vi "Configure Marker Search.vi"(0 "VISA resource name":refnum<visa-resource-name>, 1 "Search Range X (1: Full Range)":u16(ring)=1 items=["Band Marker X", "Full Range"], 2 "Peak Polarity (0: Positive)":enum16{"Positive", "Negative", "Both"}(ring), 3 "Target Transition (2: Both)":enum16{"Positive", "Negative", "Both"}(ring)=enum."Both", 5 "Measurement Type (6: Phase Noise)":u16(ring)=6 items=["AM Noise"=1, "Baseband Noise"=2, "Freq/Power"=3, "Spectrum"=4, "Transient"=5, "Phase Noise"=6, "User"=7], 7 "Select Trace (1: 1)":u16(ring)=1 items=["1"=1, "2"=2, "3"=3, "4"=4, "5"=5, "6"=6, "7"=7, "8"=8], 9 "Select Marker (1: 1)":u16(ring)=1 items=["1"=1, "2"=2, "3"=3, "4"=4, "5"=5, "6"=6, "7"=7, "8"=8, "9"=9, "10"=10], 11 "error in (no error)":errorcluster, 12 "Search Range Y (1: Full Range)":u16(ring)=1 items=["Band Marker Y", "Full Range"], 13 "Peak Excursion (0)":dbl format="%^#_9g", 14 "Target Value (0)":dbl format="%^#_9g") -> (4 "VISA resource name out":refnum<visa-resource-name>, 15 "error out":errorcluster)   [LabVIEW 2011, in "Agilent E5052X.lvlib"]
doc: "Sets the search properties for each marker in each trace.\n\n<b>Note: </b>\n\n \"Configure Marker\" VI must be run before this VI to enable markers before trying to configure their search settings."
uses:
  Agilent E5052X.lvlib
panel:
  # "Search Range Settings"
  # "Peak Search Settings"
  # "Target Search Settings"
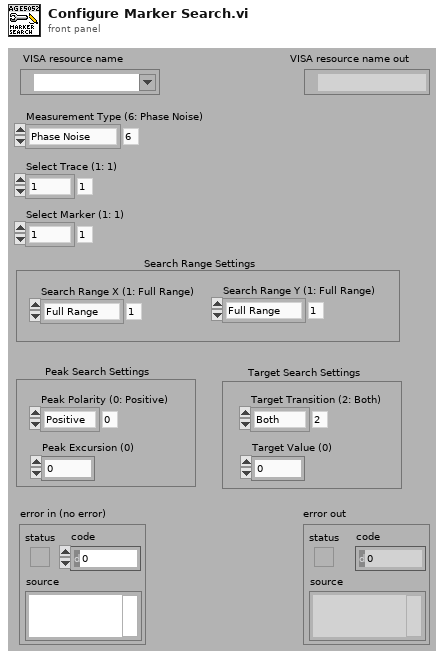
[diagram p1: front panel]
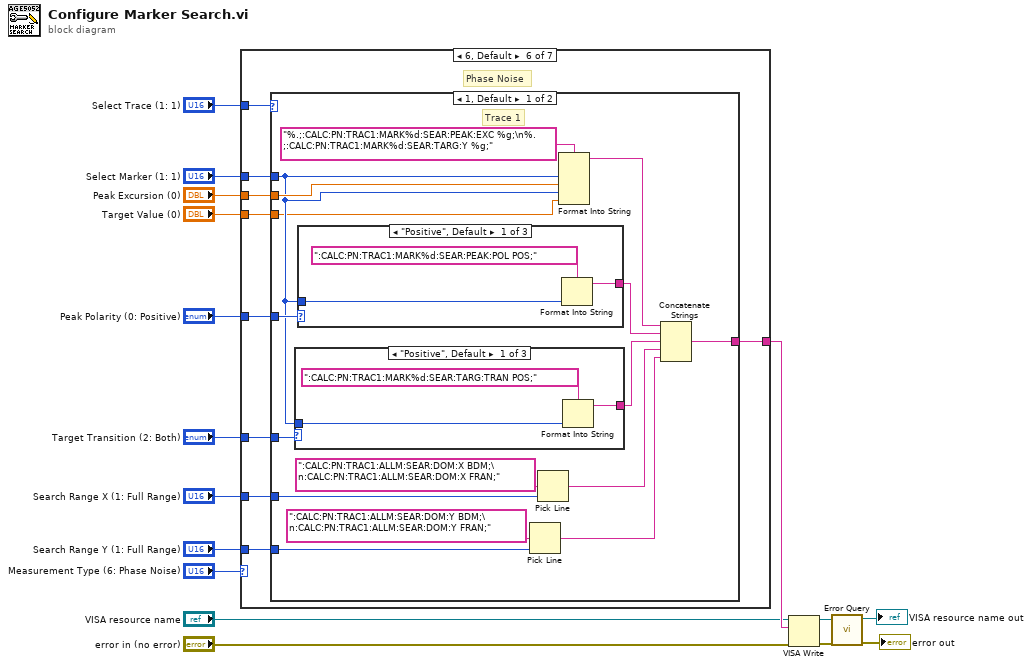
[diagram p0: block diagram]
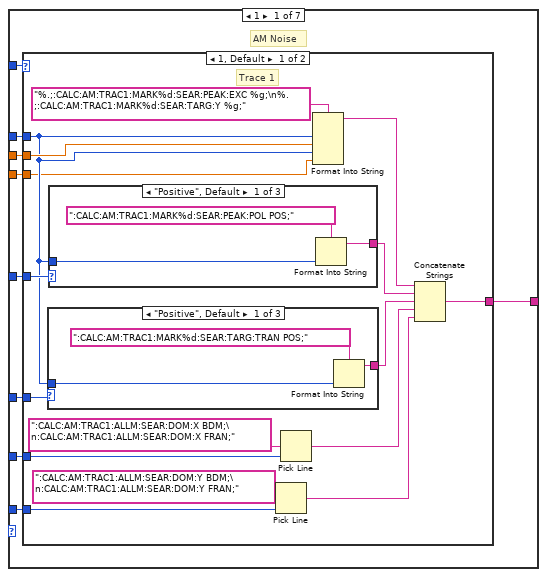
[diagram p2: hidden frame]
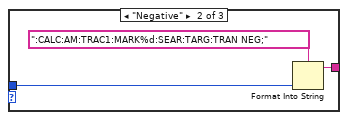
[diagram p3: hidden frame]
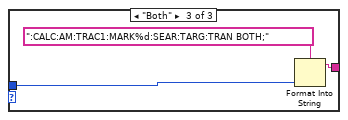
[diagram p4: hidden frame]
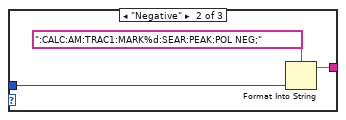
[diagram p5: hidden frame]
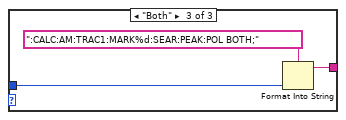
[diagram p6: hidden frame]
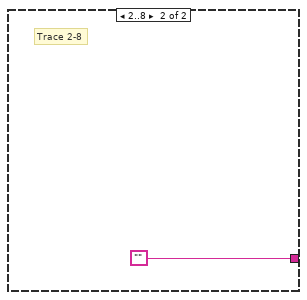
[diagram p7: hidden frame]
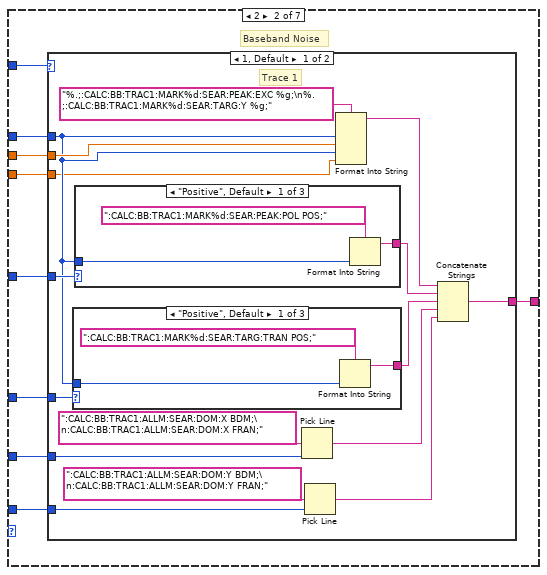
[diagram p8: hidden frame]
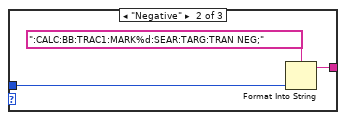
[diagram p9: hidden frame]
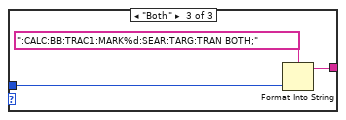
[diagram p10: hidden frame]
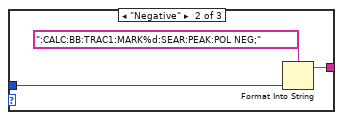
[diagram p11: hidden frame]
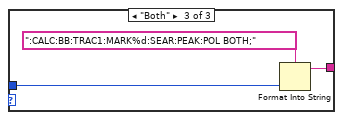
[diagram p12: hidden frame]
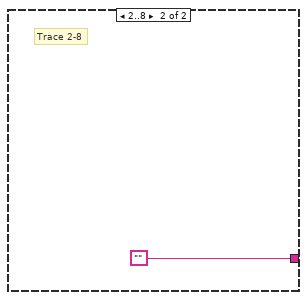
[diagram p13: hidden frame]
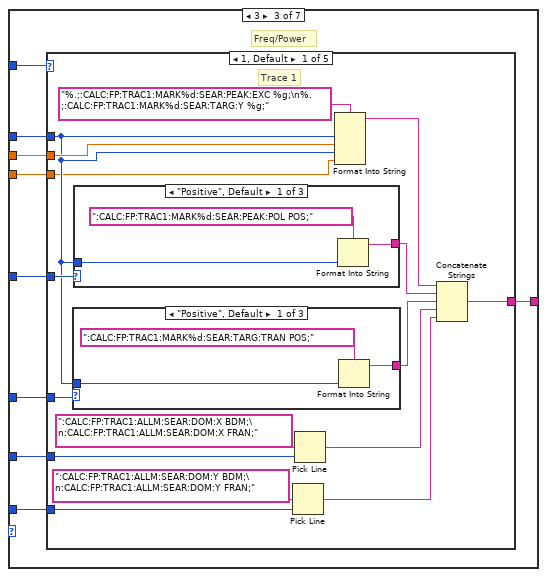
[diagram p14: hidden frame]
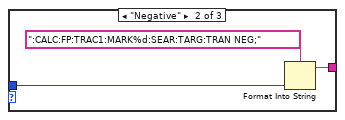
[diagram p15: hidden frame]
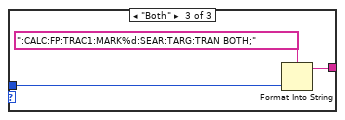
[diagram p16: hidden frame]
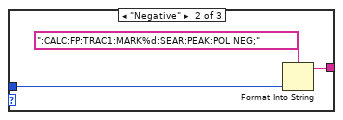
[diagram p17: hidden frame]
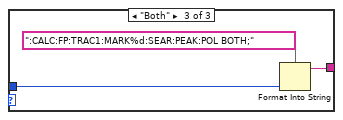
[diagram p18: hidden frame]
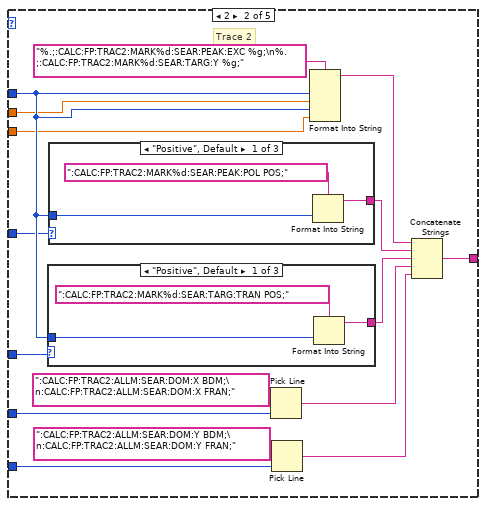
[diagram p19: hidden frame]
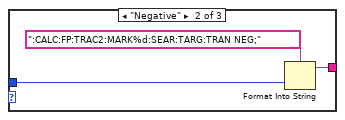
[diagram p20: hidden frame]
diagram:
  n1 = case shown="6, Default" "Measurement Type (6: Phase Noise)" {
    tunnel: "Select Marker (1: 1)" -> [w24 w68 w112 w258 w302 w448 w492]
    tunnel: "Select Trace (1: 1)" -> [w25 w69 w113 w259 w303 w449 w493]
    tunnel: "Search Range X (1: Full Range)" -> [w21 w63 w107 w253 w297 w443 w487]
    tunnel: "Search Range Y (1: Full Range)" -> [w20 w62 w106 w252 w296 w442 w486]
    tunnel: "Peak Excursion (0)" -> [w23 w67 w111 w257 w301 w447 w491]
    tunnel: "Peak Polarity (0: Positive)" -> [w22 w65 w109 w255 w299 w445 w489]
    tunnel: "Target Transition (2: Both)" -> [w19 w64 w108 w254 w298 w444 w488]
    tunnel: "Target Value (0)" -> [w18 w66 w110 w256 w300 w446 w490]
    tunnel: [w17 w61 w105 w251 w295 w441 w485] -> w8
    frame 1 {
      # "AM Noise"
      n2 = case shown="1, Default" w25 {
        tunnel: w24 -> [w37 _]
        tunnel: w23 -> [w40 _]
        tunnel: [w32 ""] -> w17
        tunnel: w22 -> [w39 _]
        tunnel: w21 -> [w30 _]
        tunnel: w20 -> [w27 _]
        tunnel: w19 -> [w38 _]
        tunnel: w18 -> [w36 _]
        frame 1, Default {
          # "Trace 1"
          n3 = case shown="\"Positive\", Default" w38 {
            tunnel: w37 -> [w44 w46 w49]
            tunnel: [w42 w45 w48] -> w33
            frame "Positive", Default {
              n4 = Format Into String(format string=":CALC:AM:TRAC1:MARK%d:SEAR:TARG:TRAN POS;", w44) -> (resulting string=w42:string)  [unwired: 2 in, 1 out]
            }
            frame "Negative" {
              n5 = Format Into String(format string=":CALC:AM:TRAC1:MARK%d:SEAR:TARG:TRAN NEG;", w46) -> (resulting string=w45:string)  [unwired: 2 in, 1 out]
            }
            frame "Both" {
              n6 = Format Into String(format string=":CALC:AM:TRAC1:MARK%d:SEAR:TARG:TRAN BOTH;", w49) -> (resulting string=w48:string)  [unwired: 2 in, 1 out]
            }
          }
          n7 = case shown="\"Positive\", Default" w39 {
            tunnel: w37 -> [w53 w55 w58]
            tunnel: [w51 w54 w57] -> w34
            frame "Positive", Default {
              n8 = Format Into String(format string=":CALC:AM:TRAC1:MARK%d:SEAR:PEAK:POL POS;", w53) -> (resulting string=w51:string)  [unwired: 2 in, 1 out]
            }
            frame "Negative" {
              n9 = Format Into String(format string=":CALC:AM:TRAC1:MARK%d:SEAR:PEAK:POL NEG;", w55) -> (resulting string=w54:string)  [unwired: 2 in, 1 out]
            }
            frame "Both" {
              n10 = Format Into String(format string=":CALC:AM:TRAC1:MARK%d:SEAR:PEAK:POL BOTH;", w58) -> (resulting string=w57:string)  [unwired: 2 in, 1 out]
            }
          }
          n11 = Pick Line(multi-line string=":CALC:AM:TRAC1:ALLM:SEAR:DOM:Y BDM;\n:CALC:AM:TRAC1:ALLM:SEAR:DOM:Y FRAN;", line index=w27) -> (output string=w26:string)  [unwired: 1 in]
          n12 = Pick Line(multi-line string=":CALC:AM:TRAC1:ALLM:SEAR:DOM:X BDM;\n:CALC:AM:TRAC1:ALLM:SEAR:DOM:X FRAN;", line index=w30) -> (output string=w29:string)  [unwired: 1 in]
          n13 = Format Into String(format string="%.;:CALC:AM:TRAC1:MARK%d:SEAR:PEAK:EXC %g;\n%.;:CALC:AM:TRAC1:MARK%d:SEAR:TARG:Y %g;", w37, w40, w37, w36) -> (resulting string=w35:string)  [unwired: 2 in, 1 out]
          n14 = Concatenate Strings(w35, w34, w33, w29, w26) -> (w32:string)
        }
        frame 2..8 {
          # "Trace 2-8"
        }
      }
    }
    frame 2 {
      # "Baseband Noise"
      n15 = case shown="1, Default" w69 {
        tunnel: w68 -> [w81 _]
        tunnel: w67 -> [w84 _]
        tunnel: [w76 ""] -> w61
        tunnel: w65 -> [w83 _]
        tunnel: w63 -> [w74 _]
        tunnel: w62 -> [w71 _]
        tunnel: w64 -> [w82 _]
        tunnel: w66 -> [w80 _]
        frame 1, Default {
          # "Trace 1"
          n16 = case shown="\"Positive\", Default" w82 {
            tunnel: w81 -> [w88 w90 w93]
            tunnel: [w86 w89 w92] -> w77
            frame "Positive", Default {
              n17 = Format Into String(format string=":CALC:BB:TRAC1:MARK%d:SEAR:TARG:TRAN POS;", w88) -> (resulting string=w86:string)  [unwired: 2 in, 1 out]
            }
            frame "Negative" {
              n18 = Format Into String(format string=":CALC:BB:TRAC1:MARK%d:SEAR:TARG:TRAN NEG;", w90) -> (resulting string=w89:string)  [unwired: 2 in, 1 out]
            }
            frame "Both" {
              n19 = Format Into String(format string=":CALC:BB:TRAC1:MARK%d:SEAR:TARG:TRAN BOTH;", w93) -> (resulting string=w92:string)  [unwired: 2 in, 1 out]
            }
          }
          n20 = case shown="\"Positive\", Default" w83 {
            tunnel: w81 -> [w97 w99 w102]
            tunnel: [w95 w98 w101] -> w78
            frame "Positive", Default {
              n21 = Format Into String(format string=":CALC:BB:TRAC1:MARK%d:SEAR:PEAK:POL POS;", w97) -> (resulting string=w95:string)  [unwired: 2 in, 1 out]
            }
            frame "Negative" {
              n22 = Format Into String(format string=":CALC:BB:TRAC1:MARK%d:SEAR:PEAK:POL NEG;", w99) -> (resulting string=w98:string)  [unwired: 2 in, 1 out]
            }
            frame "Both" {
              n23 = Format Into String(format string=":CALC:BB:TRAC1:MARK%d:SEAR:PEAK:POL BOTH;", w102) -> (resulting string=w101:string)  [unwired: 2 in, 1 out]
            }
          }
          n24 = Pick Line(multi-line string=":CALC:BB:TRAC1:ALLM:SEAR:DOM:X BDM;\n:CALC:BB:TRAC1:ALLM:SEAR:DOM:X FRAN;", line index=w74) -> (output string=w73:string)  [unwired: 1 in]
          n25 = Pick Line(multi-line string=":CALC:BB:TRAC1:ALLM:SEAR:DOM:Y BDM;\n:CALC:BB:TRAC1:ALLM:SEAR:DOM:Y FRAN;", line index=w71) -> (output string=w70:string)  [unwired: 1 in]
          n26 = Format Into String(format string="%.;:CALC:BB:TRAC1:MARK%d:SEAR:PEAK:EXC %g;\n%.;:CALC:BB:TRAC1:MARK%d:SEAR:TARG:Y %g;", w81, w84, w81, w80) -> (resulting string=w79:string)  [unwired: 2 in, 1 out]
          n27 = Concatenate Strings(w79, w78, w77, w73, w70) -> (w76:string)
        }
        frame 2..8 {
          # "Trace 2-8"
        }
      }
    }
    frame 3 {
      # "Freq/Power"
      n28 = case shown="1, Default" w113 {
        tunnel: w112 -> [w125 w159 w193 w227 _]
        tunnel: w111 -> [w128 w158 w192 w226 _]
        tunnel: [w120 w154 w188 w222 ""] -> w105
        tunnel: w109 -> [w127 w156 w190 w224 _]
        tunnel: w107 -> [w118 w152 w186 w220 _]
        tunnel: w106 -> [w115 w149 w183 w217 _]
        tunnel: w108 -> [w126 w155 w189 w223 _]
        tunnel: w110 -> [w124 w157 w191 w225 _]
        frame 1, Default {
          # "Trace 1"
          n29 = case shown="\"Positive\", Default" w126 {
            tunnel: w125 -> [w132 w134 w137]
            tunnel: [w130 w133 w136] -> w121
            frame "Positive", Default {
              n30 = Format Into String(format string=":CALC:FP:TRAC1:MARK%d:SEAR:TARG:TRAN POS;", w132) -> (resulting string=w130:string)  [unwired: 2 in, 1 out]
            }
            frame "Negative" {
              n31 = Format Into String(format string=":CALC:FP:TRAC1:MARK%d:SEAR:TARG:TRAN NEG;", w134) -> (resulting string=w133:string)  [unwired: 2 in, 1 out]
            }
            frame "Both" {
              n32 = Format Into String(format string=":CALC:FP:TRAC1:MARK%d:SEAR:TARG:TRAN BOTH;", w137) -> (resulting string=w136:string)  [unwired: 2 in, 1 out]
            }
          }
          n33 = case shown="\"Positive\", Default" w127 {
            tunnel: w125 -> [w141 w143 w146]
            tunnel: [w139 w142 w145] -> w122
            frame "Positive", Default {
              n34 = Format Into String(format string=":CALC:FP:TRAC1:MARK%d:SEAR:PEAK:POL POS;", w141) -> (resulting string=w139:string)  [unwired: 2 in, 1 out]
            }
            frame "Negative" {
              n35 = Format Into String(format string=":CALC:FP:TRAC1:MARK%d:SEAR:PEAK:POL NEG;", w143) -> (resulting string=w142:string)  [unwired: 2 in, 1 out]
            }
            frame "Both" {
              n36 = Format Into String(format string=":CALC:FP:TRAC1:MARK%d:SEAR:PEAK:POL BOTH;", w146) -> (resulting string=w145:string)  [unwired: 2 in, 1 out]
            }
          }
          n37 = Pick Line(multi-line string=":CALC:FP:TRAC1:ALLM:SEAR:DOM:Y BDM;\n:CALC:FP:TRAC1:ALLM:SEAR:DOM:Y FRAN;", line index=w115) -> (output string=w114:string)  [unwired: 1 in]
          n38 = Pick Line(multi-line string=":CALC:FP:TRAC1:ALLM:SEAR:DOM:X BDM;\n:CALC:FP:TRAC1:ALLM:SEAR:DOM:X FRAN;", line index=w118) -> (output string=w117:string)  [unwired: 1 in]
          n39 = Format Into String(format string="%.;:CALC:FP:TRAC1:MARK%d:SEAR:PEAK:EXC %g;\n%.;:CALC:FP:TRAC1:MARK%d:SEAR:TARG:Y %g;", w125, w128, w125, w124) -> (resulting string=w123:string)  [unwired: 2 in, 1 out]
          n40 = Concatenate Strings(w123, w122, w121, w117, w114) -> (w120:string)
        }
        frame 2 {
          # "Trace 2"
          n41 = case shown="\"Positive\", Default" w155 {
            tunnel: w159 -> [w166 w168 w171]
            tunnel: [w164 w167 w170] -> w160
            frame "Positive", Default {
              n42 = Format Into String(format string=":CALC:FP:TRAC2:MARK%d:SEAR:TARG:TRAN POS;", w166) -> (resulting string=w164:string)  [unwired: 2 in, 1 out]
            }
            frame "Negative" {
              n43 = Format Into String(format string=":CALC:FP:TRAC2:MARK%d:SEAR:TARG:TRAN NEG;", w168) -> (resulting string=w167:string)  [unwired: 2 in, 1 out]
            }
            frame "Both" {
              n44 = Format Into String(format string=":CALC:FP:TRAC2:MARK%d:SEAR:TARG:TRAN BOTH;", w171) -> (resulting string=w170:string)  [unwired: 2 in, 1 out]
            }
          }
          n45 = case shown="\"Positive\", Default" w156 {
            tunnel: w159 -> [w175 w177 w180]
            tunnel: [w173 w176 w179] -> w161
            frame "Positive", Default {
              n46 = Format Into String(format string=":CALC:FP:TRAC2:MARK%d:SEAR:PEAK:POL POS;", w175) -> (resulting string=w173:string)  [unwired: 2 in, 1 out]
            }
            frame "Negative" {
              n47 = Format Into String(format string=":CALC:FP:TRAC2:MARK%d:SEAR:PEAK:POL NEG;", w177) -> (resulting string=w176:string)  [unwired: 2 in, 1 out]
            }
            frame "Both" {
              n48 = Format Into String(format string=":CALC:FP:TRAC2:MARK%d:SEAR:PEAK:POL BOTH;", w180) -> (resulting string=w179:string)  [unwired: 2 in, 1 out]
            }
          }
          n49 = Pick Line(multi-line string=":CALC:FP:TRAC2:ALLM:SEAR:DOM:X BDM;\n:CALC:FP:TRAC2:ALLM:SEAR:DOM:X FRAN;", line index=w152) -> (output string=w151:string)  [unwired: 1 in]
          n50 = Pick Line(multi-line string=":CALC:FP:TRAC2:ALLM:SEAR:DOM:Y BDM;\n:CALC:FP:TRAC2:ALLM:SEAR:DOM:Y FRAN;", line index=w149) -> (output string=w148:string)  [unwired: 1 in]
          n51 = Format Into String(format string="%.;:CALC:FP:TRAC2:MARK%d:SEAR:PEAK:EXC %g;\n%.;:CALC:FP:TRAC2:MARK%d:SEAR:TARG:Y %g;", w159, w158, w159, w157) -> (resulting string=w162:string)  [unwired: 2 in, 1 out]
          n52 = Concatenate Strings(w162, w161, w160, w151, w148) -> (w154:string)
        }
        frame 3 {
          # "Trace 3"
          n53 = case shown="\"Both\"" w189 {
            tunnel: w193 -> [w200 w202 w205]
            tunnel: [w198 w201 w204] -> w194
            frame "Positive", Default {
              n54 = Format Into String(format string=":CALC:FP:TRAC3:MARK%d:SEAR:TARG:TRAN POS;", w200) -> (resulting string=w198:string)  [unwired: 2 in, 1 out]
            }
            frame "Negative" {
              n55 = Format Into String(format string=":CALC:FP:TRAC3:MARK%d:SEAR:TARG:TRAN NEG;", w202) -> (resulting string=w201:string)  [unwired: 2 in, 1 out]
            }
            frame "Both" {
              n56 = Format Into String(format string=":CALC:FP:TRAC3:MARK%d:SEAR:TARG:TRAN BOTH;", w205) -> (resulting string=w204:string)  [unwired: 2 in, 1 out]
            }
          }
          n57 = case shown="\"Positive\", Default" w190 {
            tunnel: w193 -> [w209 w211 w214]
            tunnel: [w207 w210 w213] -> w195
            frame "Positive", Default {
              n58 = Format Into String(format string=":CALC:FP:TRAC3:MARK%d:SEAR:PEAK:POL POS;", w209) -> (resulting string=w207:string)  [unwired: 2 in, 1 out]
            }
            frame "Negative" {
              n59 = Format Into String(format string=":CALC:FP:TRAC3:MARK%d:SEAR:PEAK:POL NEG;", w211) -> (resulting string=w210:string)  [unwired: 2 in, 1 out]
            }
            frame "Both" {
              n60 = Format Into String(format string=":CALC:FP:TRAC3:MARK%d:SEAR:PEAK:POL BOTH;", w214) -> (resulting string=w213:string)  [unwired: 2 in, 1 out]
            }
          }
          n61 = Pick Line(multi-line string=":CALC:FP:TRAC3:ALLM:SEAR:DOM:X BDM;\n:CALC:FP:TRAC3:ALLM:SEAR:DOM:X FRAN;", line index=w186) -> (output string=w185:string)  [unwired: 1 in]
          n62 = Pick Line(multi-line string=":CALC:FP:TRAC3:ALLM:SEAR:DOM:Y BDM;\n:CALC:FP:TRAC3:ALLM:SEAR:DOM:Y FRAN;", line index=w183) -> (output string=w182:string)  [unwired: 1 in]
          n63 = Format Into String(format string="%.;:CALC:FP:TRAC3:MARK%d:SEAR:PEAK:EXC %g;\n%.;:CALC:FP:TRAC3:MARK%d:SEAR:TARG:Y %g;", w193, w192, w193, w191) -> (resulting string=w196:string)  [unwired: 2 in, 1 out]
          n64 = Concatenate Strings(w196, w195, w194, w185, w182) -> (w188:string)
        }
        frame 4 {
          # "Trace 4"
          n65 = case shown="\"Positive\", Default" w223 {
            tunnel: w227 -> [w234 w236 w239]
            tunnel: [w232 w235 w238] -> w228
            frame "Positive", Default {
              n66 = Format Into String(format string=":CALC:FP:TRAC4:MARK%d:SEAR:TARG:TRAN POS;", w234) -> (resulting string=w232:string)  [unwired: 2 in, 1 out]
            }
            frame "Negative" {
              n67 = Format Into String(format string=":CALC:FP:TRAC4:MARK%d:SEAR:TARG:TRAN NEG;", w236) -> (resulting string=w235:string)  [unwired: 2 in, 1 out]
            }
            frame "Both" {
              n68 = Format Into String(format string=":CALC:FP:TRAC4:MARK%d:SEAR:TARG:TRAN BOTH;", w239) -> (resulting string=w238:string)  [unwired: 2 in, 1 out]
            }
          }
          n69 = case shown="\"Both\"" w224 {
            tunnel: w227 -> [w243 w245 w248]
            tunnel: [w241 w244 w247] -> w229
            frame "Positive", Default {
              n70 = Format Into String(format string=":CALC:FP:TRAC4:MARK%d:SEAR:PEAK:POL POS;", w243) -> (resulting string=w241:string)  [unwired: 2 in, 1 out]
            }
            frame "Negative" {
              n71 = Format Into String(format string=":CALC:FP:TRAC4:MARK%d:SEAR:PEAK:POL NEG;", w245) -> (resulting string=w244:string)  [unwired: 2 in, 1 out]
            }
            frame "Both" {
              n72 = Format Into String(format string=":CALC:FP:TRAC4:MARK%d:SEAR:PEAK:POL BOTH;", w248) -> (resulting string=w247:string)  [unwired: 2 in, 1 out]
            }
          }
          n73 = Pick Line(multi-line string=":CALC:FP:TRAC4:ALLM:SEAR:DOM:Y BDM;\n:CALC:FP:TRAC4:ALLM:SEAR:DOM:Y FRAN;", line index=w217) -> (output string=w216:string)  [unwired: 1 in]
          n74 = Pick Line(multi-line string=":CALC:FP:TRAC4:ALLM:SEAR:DOM:X BDM;\n:CALC:FP:TRAC4:ALLM:SEAR:DOM:X FRAN;", line index=w220) -> (output string=w219:string)  [unwired: 1 in]
          n75 = Format Into String(format string="%.;:CALC:FP:TRAC4:MARK%d:SEAR:PEAK:EXC %g;\n%.;:CALC:FP:TRAC4:MARK%d:SEAR:TARG:Y %g;", w227, w226, w227, w225) -> (resulting string=w230:string)  [unwired: 2 in, 1 out]
          n76 = Concatenate Strings(w230, w229, w228, w219, w216) -> (w222:string)
        }
        frame 5..8 {
          # "Trace 5..8"
        }
      }
    }
    frame 4 {
      # "Spectrum Monitor"
      n77 = case shown="1, Default" w259 {
        tunnel: w258 -> [w271 _]
        tunnel: w257 -> [w274 _]
        tunnel: [w266 ""] -> w251
        tunnel: w255 -> [w273 _]
        tunnel: w253 -> [w264 _]
        tunnel: w252 -> [w261 _]
        tunnel: w254 -> [w272 _]
        tunnel: w256 -> [w270 _]
        frame 1, Default {
          # "Trace 1"
          n78 = case shown="\"Positive\", Default" w272 {
            tunnel: w271 -> [w278 w280 w283]
            tunnel: [w276 w279 w282] -> w267
            frame "Positive", Default {
              n79 = Format Into String(format string=":CALC:SP:TRAC1:MARK%d:SEAR:TARG:TRAN POS;", w278) -> (resulting string=w276:string)  [unwired: 2 in, 1 out]
            }
            frame "Negative" {
              n80 = Format Into String(format string=":CALC:SP:TRAC1:MARK%d:SEAR:TARG:TRAN NEG;", w280) -> (resulting string=w279:string)  [unwired: 2 in, 1 out]
            }
            frame "Both" {
              n81 = Format Into String(format string=":CALC:SP:TRAC1:MARK%d:SEAR:TARG:TRAN BOTH;", w283) -> (resulting string=w282:string)  [unwired: 2 in, 1 out]
            }
          }
          n82 = case shown="\"Positive\", Default" w273 {
            tunnel: w271 -> [w287 w289 w292]
            tunnel: [w285 w288 w291] -> w268
            frame "Positive", Default {
              n83 = Format Into String(format string=":CALC:SP:TRAC1:MARK%d:SEAR:PEAK:POL POS;", w287) -> (resulting string=w285:string)  [unwired: 2 in, 1 out]
            }
            frame "Negative" {
              n84 = Format Into String(format string=":CALC:SP:TRAC1:MARK%d:SEAR:PEAK:POL NEG;", w289) -> (resulting string=w288:string)  [unwired: 2 in, 1 out]
            }
            frame "Both" {
              n85 = Format Into String(format string=":CALC:SP:TRAC1:MARK%d:SEAR:PEAK:POL BOTH;", w292) -> (resulting string=w291:string)  [unwired: 2 in, 1 out]
            }
          }
          n86 = Pick Line(multi-line string=":CALC:SP:TRAC1:ALLM:SEAR:DOM:X BDM;\n:CALC:SP:TRAC1:ALLM:SEAR:DOM:X FRAN;", line index=w264) -> (output string=w263:string)  [unwired: 1 in]
          n87 = Pick Line(multi-line string=":CALC:SP:TRAC1:ALLM:SEAR:DOM:Y BDM;\n:CALC:SP:TRAC1:ALLM:SEAR:DOM:Y FRAN;", line index=w261) -> (output string=w260:string)  [unwired: 1 in]
          n88 = Format Into String(format string="%.;:CALC:SP:TRAC1:MARK%d:SEAR:PEAK:EXC %g;\n%.;:CALC:SP:TRAC1:MARK%d:SEAR:TARG:Y %g;", w271, w274, w271, w270) -> (resulting string=w269:string)  [unwired: 2 in, 1 out]
          n89 = Concatenate Strings(w269, w268, w267, w263, w260) -> (w266:string)
        }
        frame 2..8 {
          # "Trace 2..8"
        }
      }
    }
    frame 5 {
      # "Transient"
      n90 = case shown="1, Default" w303 {
        tunnel: w302 -> [w315 w349 w383 w417 _]
        tunnel: w301 -> [w318 w348 w382 w416 _]
        tunnel: [w310 w344 w378 w412 ""] -> w295
        tunnel: w299 -> [w317 w346 w380 w414 _]
        tunnel: w297 -> [w308 w342 w376 w410 _]
        tunnel: w296 -> [w305 w339 w373 w407 _]
        tunnel: w298 -> [w316 w345 w379 w413 _]
        tunnel: w300 -> [w314 w347 w381 w415 _]
        frame 1, Default {
          # "Trace 1"
          n91 = case shown="\"Positive\", Default" w316 {
            tunnel: w315 -> [w322 w324 w327]
            tunnel: [w320 w323 w326] -> w311
            frame "Positive", Default {
              n92 = Format Into String(format string=":CALC:TR:TRAC1:MARK%d:SEAR:TARG:TRAN POS;", w322) -> (resulting string=w320:string)  [unwired: 2 in, 1 out]
            }
            frame "Negative" {
              n93 = Format Into String(format string=":CALC:TR:TRAC1:MARK%d:SEAR:TARG:TRAN NEG;", w324) -> (resulting string=w323:string)  [unwired: 2 in, 1 out]
            }
            frame "Both" {
              n94 = Format Into String(format string=":CALC:TR:TRAC1:MARK%d:SEAR:TARG:TRAN BOTH;", w327) -> (resulting string=w326:string)  [unwired: 2 in, 1 out]
            }
          }
          n95 = case shown="\"Positive\", Default" w317 {
            tunnel: w315 -> [w331 w333 w336]
            tunnel: [w329 w332 w335] -> w312
            frame "Positive", Default {
              n96 = Format Into String(format string=":CALC:TR:TRAC1:MARK%d:SEAR:PEAK:POL POS;", w331) -> (resulting string=w329:string)  [unwired: 2 in, 1 out]
            }
            frame "Negative" {
              n97 = Format Into String(format string=":CALC:TR:TRAC1:MARK%d:SEAR:PEAK:POL NEG;", w333) -> (resulting string=w332:string)  [unwired: 2 in, 1 out]
            }
            frame "Both" {
              n98 = Format Into String(format string=":CALC:TR:TRAC1:MARK%d:SEAR:PEAK:POL BOTH;", w336) -> (resulting string=w335:string)  [unwired: 2 in, 1 out]
            }
          }
          n99 = Pick Line(multi-line string=":CALC:TR:TRAC1:ALLM:SEAR:DOM:X BDM;\n:CALC:TR:TRAC1:ALLM:SEAR:DOM:X FRAN;", line index=w308) -> (output string=w307:string)  [unwired: 1 in]
          n100 = Pick Line(multi-line string=":CALC:TR:TRAC1:ALLM:SEAR:DOM:Y BDM;\n:CALC:TR:TRAC1:ALLM:SEAR:DOM:Y FRAN;", line index=w305) -> (output string=w304:string)  [unwired: 1 in]
          n101 = Format Into String(format string="%.;:CALC:TR:TRAC1:MARK%d:SEAR:PEAK:EXC %g;\n%.;:CALC:TR:TRAC1:MARK%d:SEAR:TARG:Y %g;", w315, w318, w315, w314) -> (resulting string=w313:string)  [unwired: 2 in, 1 out]
          n102 = Concatenate Strings(w313, w312, w311, w307, w304) -> (w310:string)
        }
        frame 2 {
          # "Trace 2"
          n103 = case shown="\"Both\"" w345 {
            tunnel: w349 -> [w356 w358 w361]
            tunnel: [w354 w357 w360] -> w350
            frame "Positive", Default {
              n104 = Format Into String(format string=":CALC:TR:TRAC2:MARK%d:SEAR:TARG:TRAN POS;", w356) -> (resulting string=w354:string)  [unwired: 2 in, 1 out]
            }
            frame "Negative" {
              n105 = Format Into String(format string=":CALC:TR:TRAC2:MARK%d:SEAR:TARG:TRAN NEG;", w358) -> (resulting string=w357:string)  [unwired: 2 in, 1 out]
            }
            frame "Both" {
              n106 = Format Into String(format string=":CALC:TR:TRAC2:MARK%d:SEAR:TARG:TRAN BOTH;", w361) -> (resulting string=w360:string)  [unwired: 2 in, 1 out]
            }
          }
          n107 = case shown="\"Negative\"" w346 {
            tunnel: w349 -> [w365 w367 w370]
            tunnel: [w363 w366 w369] -> w351
            frame "Positive", Default {
              n108 = Format Into String(format string=":CALC:TR:TRAC2:MARK%d:SEAR:PEAK:POL POS;", w365) -> (resulting string=w363:string)  [unwired: 2 in, 1 out]
            }
            frame "Negative" {
              n109 = Format Into String(format string=":CALC:TR:TRAC2:MARK%d:SEAR:PEAK:POL NEG;", w367) -> (resulting string=w366:string)  [unwired: 2 in, 1 out]
            }
            frame "Both" {
              n110 = Format Into String(format string=":CALC:TR:TRAC2:MARK%d:SEAR:PEAK:POL BOTH;", w370) -> (resulting string=w369:string)  [unwired: 2 in, 1 out]
            }
          }
          n111 = Pick Line(multi-line string=":CALC:TR:TRAC2:ALLM:SEAR:DOM:X BDM;\n:CALC:TR:TRAC2:ALLM:SEAR:DOM:X FRAN;", line index=w342) -> (output string=w341:string)  [unwired: 1 in]
          n112 = Pick Line(multi-line string=":CALC:TR:TRAC2:ALLM:SEAR:DOM:Y BDM;\n:CALC:TR:TRAC2:ALLM:SEAR:DOM:Y FRAN;", line index=w339) -> (output string=w338:string)  [unwired: 1 in]
          n113 = Format Into String(format string="%.;:CALC:TR:TRAC2:MARK%d:SEAR:PEAK:EXC %g;\n%.;:CALC:TR:TRAC2:MARK%d:SEAR:TARG:Y %g;", w349, w348, w349, w347) -> (resulting string=w352:string)  [unwired: 2 in, 1 out]
          n114 = Concatenate Strings(w352, w351, w350, w341, w338) -> (w344:string)
        }
        frame 3 {
          # "Trace 3"
          n115 = case shown="\"Positive\", Default" w379 {
            tunnel: w383 -> [w390 w392 w395]
            tunnel: [w388 w391 w394] -> w384
            frame "Positive", Default {
              n116 = Format Into String(format string=":CALC:TR:TRAC3:MARK%d:SEAR:TARG:TRAN POS;", w390) -> (resulting string=w388:string)  [unwired: 2 in, 1 out]
            }
            frame "Negative" {
              n117 = Format Into String(format string=":CALC:TR:TRAC3:MARK%d:SEAR:TARG:TRAN NEG;", w392) -> (resulting string=w391:string)  [unwired: 2 in, 1 out]
            }
            frame "Both" {
              n118 = Format Into String(format string=":CALC:TR:TRAC3:MARK%d:SEAR:TARG:TRAN BOTH;", w395) -> (resulting string=w394:string)  [unwired: 2 in, 1 out]
            }
          }
          n119 = case shown="\"Positive\", Default" w380 {
            tunnel: w383 -> [w399 w401 w404]
            tunnel: [w397 w400 w403] -> w385
            frame "Positive", Default {
              n120 = Format Into String(format string=":CALC:TR:TRAC3:MARK%d:SEAR:PEAK:POL POS;", w399) -> (resulting string=w397:string)  [unwired: 2 in, 1 out]
            }
            frame "Negative" {
              n121 = Format Into String(format string=":CALC:TR:TRAC3:MARK%d:SEAR:PEAK:POL NEG;", w401) -> (resulting string=w400:string)  [unwired: 2 in, 1 out]
            }
            frame "Both" {
              n122 = Format Into String(format string=":CALC:TR:TRAC3:MARK%d:SEAR:PEAK:POL BOTH;", w404) -> (resulting string=w403:string)  [unwired: 2 in, 1 out]
            }
          }
          n123 = Pick Line(multi-line string=":CALC:TR:TRAC3:ALLM:SEAR:DOM:Y BDM;\n:CALC:TR:TRAC3:ALLM:SEAR:DOM:Y FRAN;", line index=w373) -> (output string=w372:string)  [unwired: 1 in]
          n124 = Pick Line(multi-line string=":CALC:TR:TRAC3:ALLM:SEAR:DOM:X BDM;\n:CALC:TR:TRAC3:ALLM:SEAR:DOM:X FRAN;", line index=w376) -> (output string=w375:string)  [unwired: 1 in]
          n125 = Format Into String(format string="%.;:CALC:TR:TRAC3:MARK%d:SEAR:PEAK:EXC %g;\n%.;:CALC:TR:TRAC3:MARK%d:SEAR:TARG:Y %g;", w383, w382, w383, w381) -> (resulting string=w386:string)  [unwired: 2 in, 1 out]
          n126 = Concatenate Strings(w386, w385, w384, w375, w372) -> (w378:string)
        }
        frame 4 {
          # "Trace 4"
          n127 = case shown="\"Positive\", Default" w413 {
            tunnel: w417 -> [w424 w426 w429]
            tunnel: [w422 w425 w428] -> w418
            frame "Positive", Default {
              n128 = Format Into String(format string=":CALC:TR:TRAC4:MARK%d:SEAR:TARG:TRAN POS;", w424) -> (resulting string=w422:string)  [unwired: 2 in, 1 out]
            }
            frame "Negative" {
              n129 = Format Into String(format string=":CALC:TR:TRAC4:MARK%d:SEAR:TARG:TRAN NEG;", w426) -> (resulting string=w425:string)  [unwired: 2 in, 1 out]
            }
            frame "Both" {
              n130 = Format Into String(format string=":CALC:TR:TRAC4:MARK%d:SEAR:TARG:TRAN BOTH;", w429) -> (resulting string=w428:string)  [unwired: 2 in, 1 out]
            }
          }
          n131 = case shown="\"Positive\", Default" w414 {
            tunnel: w417 -> [w433 w435 w438]
            tunnel: [w431 w434 w437] -> w419
            frame "Positive", Default {
              n132 = Format Into String(format string=":CALC:TR:TRAC4:MARK%d:SEAR:PEAK:POL POS;", w433) -> (resulting string=w431:string)  [unwired: 2 in, 1 out]
            }
            frame "Negative" {
              n133 = Format Into String(format string=":CALC:TR:TRAC4:MARK%d:SEAR:PEAK:POL NEG;", w435) -> (resulting string=w434:string)  [unwired: 2 in, 1 out]
            }
            frame "Both" {
              n134 = Format Into String(format string=":CALC:TR:TRAC4:MARK%d:SEAR:PEAK:POL BOTH;", w438) -> (resulting string=w437:string)  [unwired: 2 in, 1 out]
            }
          }
          n135 = Pick Line(multi-line string=":CALC:TR:TRAC4:ALLM:SEAR:DOM:Y BDM;\n:CALC:TR:TRAC4:ALLM:SEAR:DOM:Y FRAN;", line index=w407) -> (output string=w406:string)  [unwired: 1 in]
          n136 = Pick Line(multi-line string=":CALC:TR:TRAC4:ALLM:SEAR:DOM:X BDM;\n:CALC:TR:TRAC4:ALLM:SEAR:DOM:X FRAN;", line index=w410) -> (output string=w409:string)  [unwired: 1 in]
          n137 = Format Into String(format string="%.;:CALC:TR:TRAC4:MARK%d:SEAR:PEAK:EXC %g;\n%.;:CALC:TR:TRAC4:MARK%d:SEAR:TARG:Y %g;", w417, w416, w417, w415) -> (resulting string=w420:string)  [unwired: 2 in, 1 out]
          n138 = Concatenate Strings(w420, w419, w418, w409, w406) -> (w412:string)
        }
        frame 5..8 {
          # "Trace 5..8"
        }
      }
    }
    frame 6, Default {
      # "Phase Noise"
      n139 = case shown="1, Default" w449 {
        tunnel: w448 -> [w461 _]
        tunnel: w447 -> [w464 _]
        tunnel: [w456 ""] -> w441
        tunnel: w445 -> [w463 _]
        tunnel: w443 -> [w454 _]
        tunnel: w442 -> [w451 _]
        tunnel: w444 -> [w462 _]
        tunnel: w446 -> [w460 _]
        frame 1, Default {
          # "Trace 1"
          n140 = case shown="\"Positive\", Default" w462 {
            tunnel: w461 -> [w468 w470 w473]
            tunnel: [w466 w469 w472] -> w457
            frame "Positive", Default {
              n141 = Format Into String(format string=":CALC:PN:TRAC1:MARK%d:SEAR:TARG:TRAN POS;", w468) -> (resulting string=w466:string)  [unwired: 2 in, 1 out]
            }
            frame "Negative" {
              n142 = Format Into String(format string=":CALC:PN:TRAC1:MARK%d:SEAR:TARG:TRAN NEG;", w470) -> (resulting string=w469:string)  [unwired: 2 in, 1 out]
            }
            frame "Both" {
              n143 = Format Into String(format string=":CALC:PN:TRAC1:MARK%d:SEAR:TARG:TRAN BOTH;", w473) -> (resulting string=w472:string)  [unwired: 2 in, 1 out]
            }
          }
          n144 = case shown="\"Positive\", Default" w463 {
            tunnel: w461 -> [w477 w479 w482]
            tunnel: [w475 w478 w481] -> w458
            frame "Positive", Default {
              n145 = Format Into String(format string=":CALC:PN:TRAC1:MARK%d:SEAR:PEAK:POL POS;", w477) -> (resulting string=w475:string)  [unwired: 2 in, 1 out]
            }
            frame "Negative" {
              n146 = Format Into String(format string=":CALC:PN:TRAC1:MARK%d:SEAR:PEAK:POL NEG;", w479) -> (resulting string=w478:string)  [unwired: 2 in, 1 out]
            }
            frame "Both" {
              n147 = Format Into String(format string=":CALC:PN:TRAC1:MARK%d:SEAR:PEAK:POL BOTH;", w482) -> (resulting string=w481:string)  [unwired: 2 in, 1 out]
            }
          }
          n148 = Pick Line(multi-line string=":CALC:PN:TRAC1:ALLM:SEAR:DOM:Y BDM;\n:CALC:PN:TRAC1:ALLM:SEAR:DOM:Y FRAN;", line index=w451) -> (output string=w450:string)  [unwired: 1 in]
          n149 = Pick Line(multi-line string=":CALC:PN:TRAC1:ALLM:SEAR:DOM:X BDM;\n:CALC:PN:TRAC1:ALLM:SEAR:DOM:X FRAN;", line index=w454) -> (output string=w453:string)  [unwired: 1 in]
          n150 = Format Into String(format string="%.;:CALC:PN:TRAC1:MARK%d:SEAR:PEAK:EXC %g;\n%.;:CALC:PN:TRAC1:MARK%d:SEAR:TARG:Y %g;", w461, w464, w461, w460) -> (resulting string=w459:string)  [unwired: 2 in, 1 out]
          n151 = Concatenate Strings(w459, w458, w457, w453, w450) -> (w456:string)
        }
        frame 2..8 {
          # "Trace 2-8"
        }
      }
    }
    frame 7 {
      # "User"
      n152 = case shown="1, Default" w493 {
        tunnel: w492 -> [w505 w539 w573 w607 w641 w674 w709 w743]
        tunnel: w491 -> [w508 w538 w572 w606 w640 w673 w708 w742]
        tunnel: [w500 w534 w568 w602 w636 w675 w704 w738] -> w485
        tunnel: w489 -> [w507 w536 w570 w604 w638 w671 w706 w740]
        tunnel: w487 -> [w498 w532 w566 w600 w634 w668 w702 w736]
        tunnel: w486 -> [w495 w529 w563 w597 w631 w665 w699 w733]
        tunnel: w488 -> [w506 w535 w569 w603 w637 w670 w705 w739]
        tunnel: w490 -> [w504 w537 w571 w605 w639 w672 w707 w741]
        frame 1, Default {
          # "Trace 1"
          n153 = case shown="\"Positive\", Default" w506 {
            tunnel: w505 -> [w512 w514 w517]
            tunnel: [w510 w513 w516] -> w501
            frame "Positive", Default {
              n154 = Format Into String(format string=":CALC:USER:TRAC1:MARK%d:SEAR:TARG:TRAN POS;", w512) -> (resulting string=w510:string)  [unwired: 2 in, 1 out]
            }
            frame "Negative" {
              n155 = Format Into String(format string=":CALC:USER:TRAC1:MARK%d:SEAR:TARG:TRAN NEG;", w514) -> (resulting string=w513:string)  [unwired: 2 in, 1 out]
            }
            frame "Both" {
              n156 = Format Into String(format string=":CALC:USER:TRAC1:MARK%d:SEAR:TARG:TRAN BOTH;", w517) -> (resulting string=w516:string)  [unwired: 2 in, 1 out]
            }
          }
          n157 = case shown="\"Positive\", Default" w507 {
            tunnel: w505 -> [w521 w523 w526]
            tunnel: [w519 w522 w525] -> w502
            frame "Positive", Default {
              n158 = Format Into String(format string=":CALC:USER:TRAC1:MARK%d:SEAR:PEAK:POL POS;", w521) -> (resulting string=w519:string)  [unwired: 2 in, 1 out]
            }
            frame "Negative" {
              n159 = Format Into String(format string=":CALC:USER:TRAC1:MARK%d:SEAR:PEAK:POL NEG;", w523) -> (resulting string=w522:string)  [unwired: 2 in, 1 out]
            }
            frame "Both" {
              n160 = Format Into String(format string=":CALC:USER:TRAC1:MARK%d:SEAR:PEAK:POL BOTH;", w526) -> (resulting string=w525:string)  [unwired: 2 in, 1 out]
            }
          }
          n161 = Pick Line(multi-line string=":CALC:USER:TRAC1:ALLM:SEAR:DOM:X BDM;\n:CALC:USER:TRAC1:ALLM:SEAR:DOM:X FRAN;", line index=w498) -> (output string=w497:string)  [unwired: 1 in]
          n162 = Pick Line(multi-line string=":CALC:USER:TRAC1:ALLM:SEAR:DOM:Y BDM;\n:CALC:USER:TRAC1:ALLM:SEAR:DOM:Y FRAN;", line index=w495) -> (output string=w494:string)  [unwired: 1 in]
          n163 = Format Into String(format string="%.;:CALC:USER:TRAC1:MARK%d:SEAR:PEAK:EXC %g;\n%.;:CALC:USER:TRAC1:MARK%d:SEAR:TARG:Y %g;", w505, w508, w505, w504) -> (resulting string=w503:string)  [unwired: 2 in, 1 out]
          n164 = Concatenate Strings(w503, w502, w501, w497, w494) -> (w500:string)
        }
        frame 2 {
          # "Trace 2"
          n165 = case shown="\"Positive\", Default" w535 {
            tunnel: w539 -> [w546 w548 w551]
            tunnel: [w544 w547 w550] -> w540
            frame "Positive", Default {
              n166 = Format Into String(format string=":CALC:USER:TRAC2:MARK%d:SEAR:TARG:TRAN POS;", w546) -> (resulting string=w544:string)  [unwired: 2 in, 1 out]
            }
            frame "Negative" {
              n167 = Format Into String(format string=":CALC:USER:TRAC2:MARK%d:SEAR:TARG:TRAN NEG;", w548) -> (resulting string=w547:string)  [unwired: 2 in, 1 out]
            }
            frame "Both" {
              n168 = Format Into String(format string=":CALC:USER:TRAC2:MARK%d:SEAR:TARG:TRAN BOTH;", w551) -> (resulting string=w550:string)  [unwired: 2 in, 1 out]
            }
          }
          n169 = case shown="\"Positive\", Default" w536 {
            tunnel: w539 -> [w555 w557 w560]
            tunnel: [w553 w556 w559] -> w541
            frame "Positive", Default {
              n170 = Format Into String(format string=":CALC:USER:TRAC2:MARK%d:SEAR:PEAK:POL POS;", w555) -> (resulting string=w553:string)  [unwired: 2 in, 1 out]
            }
            frame "Negative" {
              n171 = Format Into String(format string=":CALC:USER:TRAC2:MARK%d:SEAR:PEAK:POL NEG;", w557) -> (resulting string=w556:string)  [unwired: 2 in, 1 out]
            }
            frame "Both" {
              n172 = Format Into String(format string=":CALC:USER:TRAC2:MARK%d:SEAR:PEAK:POL BOTH;", w560) -> (resulting string=w559:string)  [unwired: 2 in, 1 out]
            }
          }
          n173 = Pick Line(multi-line string=":CALC:USER:TRAC2:ALLM:SEAR:DOM:X BDM;\n:CALC:USER:TRAC2:ALLM:SEAR:DOM:X FRAN;", line index=w532) -> (output string=w531:string)  [unwired: 1 in]
          n174 = Pick Line(multi-line string=":CALC:USER:TRAC2:ALLM:SEAR:DOM:Y BDM;\n:CALC:USER:TRAC2:ALLM:SEAR:DOM:Y FRAN;", line index=w529) -> (output string=w528:string)  [unwired: 1 in]
          n175 = Format Into String(format string="%.;:CALC:USER:TRAC2:MARK%d:SEAR:PEAK:EXC %g;\n%.;:CALC:USER:TRAC2:MARK%d:SEAR:TARG:Y %g;", w539, w538, w539, w537) -> (resulting string=w542:string)  [unwired: 2 in, 1 out]
          n176 = Concatenate Strings(w542, w541, w540, w531, w528) -> (w534:string)
        }
        frame 3 {
          # "Trace 3"
          n177 = case shown="\"Positive\", Default" w569 {
            tunnel: w573 -> [w580 w582 w585]
            tunnel: [w578 w581 w584] -> w574
            frame "Positive", Default {
              n178 = Format Into String(format string=":CALC:USER:TRAC3:MARK%d:SEAR:TARG:TRAN POS;", w580) -> (resulting string=w578:string)  [unwired: 2 in, 1 out]
            }
            frame "Negative" {
              n179 = Format Into String(format string=":CALC:USER:TRAC3:MARK%d:SEAR:TARG:TRAN NEG;", w582) -> (resulting string=w581:string)  [unwired: 2 in, 1 out]
            }
            frame "Both" {
              n180 = Format Into String(format string=":CALC:USER:TRAC3:MARK%d:SEAR:TARG:TRAN BOTH;", w585) -> (resulting string=w584:string)  [unwired: 2 in, 1 out]
            }
          }
          n181 = case shown="\"Positive\", Default" w570 {
            tunnel: w573 -> [w589 w591 w594]
            tunnel: [w587 w590 w593] -> w575
            frame "Positive", Default {
              n182 = Format Into String(format string=":CALC:USER:TRAC3:MARK%d:SEAR:PEAK:POL POS;", w589) -> (resulting string=w587:string)  [unwired: 2 in, 1 out]
            }
            frame "Negative" {
              n183 = Format Into String(format string=":CALC:USER:TRAC3:MARK%d:SEAR:PEAK:POL NEG;", w591) -> (resulting string=w590:string)  [unwired: 2 in, 1 out]
            }
            frame "Both" {
              n184 = Format Into String(format string=":CALC:USER:TRAC3:MARK%d:SEAR:PEAK:POL BOTH;", w594) -> (resulting string=w593:string)  [unwired: 2 in, 1 out]
            }
          }
          n185 = Pick Line(multi-line string=":CALC:USER:TRAC3:ALLM:SEAR:DOM:X BDM;\n:CALC:USER:TRAC3:ALLM:SEAR:DOM:X FRAN;", line index=w566) -> (output string=w565:string)  [unwired: 1 in]
          n186 = Pick Line(multi-line string=":CALC:USER:TRAC3:ALLM:SEAR:DOM:Y BDM;\n:CALC:USER:TRAC3:ALLM:SEAR:DOM:Y FRAN;", line index=w563) -> (output string=w562:string)  [unwired: 1 in]
          n187 = Format Into String(format string="%.;:CALC:USER:TRAC3:MARK%d:SEAR:PEAK:EXC %g;\n%.;:CALC:USER:TRAC3:MARK%d:SEAR:TARG:Y %g;", w573, w572, w573, w571) -> (resulting string=w576:string)  [unwired: 2 in, 1 out]
          n188 = Concatenate Strings(w576, w575, w574, w565, w562) -> (w568:string)
        }
        frame 4 {
          # "Trace 4"
          n189 = case shown="\"Positive\", Default" w603 {
            tunnel: w607 -> [w614 w616 w619]
            tunnel: [w612 w615 w618] -> w608
            frame "Positive", Default {
              n190 = Format Into String(format string=":CALC:USER:TRAC4:MARK%d:SEAR:TARG:TRAN POS;", w614) -> (resulting string=w612:string)  [unwired: 2 in, 1 out]
            }
            frame "Negative" {
              n191 = Format Into String(format string=":CALC:USER:TRAC4:MARK%d:SEAR:TARG:TRAN NEG;", w616) -> (resulting string=w615:string)  [unwired: 2 in, 1 out]
            }
            frame "Both" {
              n192 = Format Into String(format string=":CALC:USER:TRAC4:MARK%d:SEAR:TARG:TRAN BOTH;", w619) -> (resulting string=w618:string)  [unwired: 2 in, 1 out]
            }
          }
          n193 = case shown="\"Positive\", Default" w604 {
            tunnel: w607 -> [w623 w625 w628]
            tunnel: [w621 w624 w627] -> w609
            frame "Positive", Default {
              n194 = Format Into String(format string=":CALC:USER:TRAC4:MARK%d:SEAR:PEAK:POL POS;", w623) -> (resulting string=w621:string)  [unwired: 2 in, 1 out]
            }
            frame "Negative" {
              n195 = Format Into String(format string=":CALC:USER:TRAC4:MARK%d:SEAR:PEAK:POL NEG;", w625) -> (resulting string=w624:string)  [unwired: 2 in, 1 out]
            }
            frame "Both" {
              n196 = Format Into String(format string=":CALC:USER:TRAC4:MARK%d:SEAR:PEAK:POL BOTH;", w628) -> (resulting string=w627:string)  [unwired: 2 in, 1 out]
            }
          }
          n197 = Pick Line(multi-line string=":CALC:USER:TRAC4:ALLM:SEAR:DOM:Y BDM;\n:CALC:USER:TRAC4:ALLM:SEAR:DOM:Y FRAN;", line index=w597) -> (output string=w596:string)  [unwired: 1 in]
          n198 = Pick Line(multi-line string=":CALC:USER:TRAC4:ALLM:SEAR:DOM:X BDM;\n:CALC:USER:TRAC4:ALLM:SEAR:DOM:X FRAN;", line index=w600) -> (output string=w599:string)  [unwired: 1 in]
          n199 = Format Into String(format string="%.;:CALC:USER:TRAC4:MARK%d:SEAR:PEAK:EXC %g;\n%.;:CALC:USER:TRAC4:MARK%d:SEAR:TARG:Y %g;", w607, w606, w607, w605) -> (resulting string=w610:string)  [unwired: 2 in, 1 out]
          n200 = Concatenate Strings(w610, w609, w608, w599, w596) -> (w602:string)
        }
        frame 5 {
          # "Trace 5"
          n201 = case shown="\"Positive\", Default" w637 {
            tunnel: w641 -> [w648 w650 w653]
            tunnel: [w646 w649 w652] -> w642
            frame "Positive", Default {
              n202 = Format Into String(format string=":CALC:USER:TRAC5:MARK%d:SEAR:TARG:TRAN POS;", w648) -> (resulting string=w646:string)  [unwired: 2 in, 1 out]
            }
            frame "Negative" {
              n203 = Format Into String(format string=":CALC:USER:TRAC5:MARK%d:SEAR:TARG:TRAN NEG;", w650) -> (resulting string=w649:string)  [unwired: 2 in, 1 out]
            }
            frame "Both" {
              n204 = Format Into String(format string=":CALC:USER:TRAC5:MARK%d:SEAR:TARG:TRAN BOTH;", w653) -> (resulting string=w652:string)  [unwired: 2 in, 1 out]
            }
          }
          n205 = case shown="\"Positive\", Default" w638 {
            tunnel: w641 -> [w657 w659 w662]
            tunnel: [w655 w658 w661] -> w643
            frame "Positive", Default {
              n206 = Format Into String(format string=":CALC:USER:TRAC5:MARK%d:SEAR:PEAK:POL POS;", w657) -> (resulting string=w655:string)  [unwired: 2 in, 1 out]
            }
            frame "Negative" {
              n207 = Format Into String(format string=":CALC:USER:TRAC5:MARK%d:SEAR:PEAK:POL NEG;", w659) -> (resulting string=w658:string)  [unwired: 2 in, 1 out]
            }
            frame "Both" {
              n208 = Format Into String(format string=":CALC:USER:TRAC5:MARK%d:SEAR:PEAK:POL BOTH;", w662) -> (resulting string=w661:string)  [unwired: 2 in, 1 out]
            }
          }
          n209 = Pick Line(multi-line string=":CALC:USER:TRAC5:ALLM:SEAR:DOM:X BDM;\n:CALC:USER:TRAC5:ALLM:SEAR:DOM:X FRAN;", line index=w634) -> (output string=w633:string)  [unwired: 1 in]
          n210 = Pick Line(multi-line string=":CALC:USER:TRAC5:ALLM:SEAR:DOM:Y BDM;\n:CALC:USER:TRAC5:ALLM:SEAR:DOM:Y FRAN;", line index=w631) -> (output string=w630:string)  [unwired: 1 in]
          n211 = Format Into String(format string="%.;:CALC:USER:TRAC5:MARK%d:SEAR:PEAK:EXC %g;\n%.;:CALC:USER:TRAC5:MARK%d:SEAR:TARG:Y %g;", w641, w640, w641, w639) -> (resulting string=w644:string)  [unwired: 2 in, 1 out]
          n212 = Concatenate Strings(w644, w643, w642, w633, w630) -> (w636:string)
        }
        frame 6 {
          # "Trace 6"
          n213 = case shown="\"Positive\", Default" w670 {
            tunnel: w674 -> [w682 w684 w687]
            tunnel: [w680 w683 w686] -> w676
            frame "Positive", Default {
              n214 = Format Into String(format string=":CALC:USER:TRAC6:MARK%d:SEAR:TARG:TRAN POS;", w682) -> (resulting string=w680:string)  [unwired: 2 in, 1 out]
            }
            frame "Negative" {
              n215 = Format Into String(format string=":CALC:USER:TRAC6:MARK%d:SEAR:TARG:TRAN NEG;", w684) -> (resulting string=w683:string)  [unwired: 2 in, 1 out]
            }
            frame "Both" {
              n216 = Format Into String(format string=":CALC:USER:TRAC6:MARK%d:SEAR:TARG:TRAN BOTH;", w687) -> (resulting string=w686:string)  [unwired: 2 in, 1 out]
            }
          }
          n217 = case shown="\"Positive\", Default" w671 {
            tunnel: w674 -> [w691 w693 w696]
            tunnel: [w689 w692 w695] -> w677
            frame "Positive", Default {
              n218 = Format Into String(format string=":CALC:USER:TRAC6:MARK%d:SEAR:PEAK:POL POS;", w691) -> (resulting string=w689:string)  [unwired: 2 in, 1 out]
            }
            frame "Negative" {
              n219 = Format Into String(format string=":CALC:USER:TRAC6:MARK%d:SEAR:PEAK:POL NEG;", w693) -> (resulting string=w692:string)  [unwired: 2 in, 1 out]
            }
            frame "Both" {
              n220 = Format Into String(format string=":CALC:USER:TRAC6:MARK%d:SEAR:PEAK:POL BOTH;", w696) -> (resulting string=w695:string)  [unwired: 2 in, 1 out]
            }
          }
          n221 = Pick Line(multi-line string=":CALC:USER:TRAC6:ALLM:SEAR:DOM:Y BDM;\n:CALC:USER:TRAC6:ALLM:SEAR:DOM:Y FRAN;", line index=w665) -> (output string=w664:string)  [unwired: 1 in]
          n222 = Pick Line(multi-line string=":CALC:USER:TRAC6:ALLM:SEAR:DOM:X BDM;\n:CALC:USER:TRAC6:ALLM:SEAR:DOM:X FRAN;", line index=w668) -> (output string=w667:string)  [unwired: 1 in]
          n223 = Format Into String(format string="%.;:CALC:USER:TRAC6:MARK%d:SEAR:PEAK:EXC %g;\n%.;:CALC:USER:TRAC6:MARK%d:SEAR:TARG:Y %g;", w674, w673, w674, w672) -> (resulting string=w678:string)  [unwired: 2 in, 1 out]
          n224 = Concatenate Strings(w678, w677, w676, w667, w664) -> (w675:string)
        }
        frame 7 {
          # "Trace 7"
          n225 = case shown="\"Positive\", Default" w705 {
            tunnel: w709 -> [w716 w718 w721]
            tunnel: [w714 w717 w720] -> w710
            frame "Positive", Default {
              n226 = Format Into String(format string=":CALC:USER:TRAC7:MARK%d:SEAR:TARG:TRAN POS;", w716) -> (resulting string=w714:string)  [unwired: 2 in, 1 out]
            }
            frame "Negative" {
              n227 = Format Into String(format string=":CALC:USER:TRAC7:MARK%d:SEAR:TARG:TRAN NEG;", w718) -> (resulting string=w717:string)  [unwired: 2 in, 1 out]
            }
            frame "Both" {
              n228 = Format Into String(format string=":CALC:USER:TRAC7:MARK%d:SEAR:TARG:TRAN BOTH;", w721) -> (resulting string=w720:string)  [unwired: 2 in, 1 out]
            }
          }
          n229 = case shown="\"Positive\", Default" w706 {
            tunnel: w709 -> [w725 w727 w730]
            tunnel: [w723 w726 w729] -> w711
            frame "Positive", Default {
              n230 = Format Into String(format string=":CALC:USER:TRAC7:MARK%d:SEAR:PEAK:POL POS;", w725) -> (resulting string=w723:string)  [unwired: 2 in, 1 out]
            }
            frame "Negative" {
              n231 = Format Into String(format string=":CALC:USER:TRAC7:MARK%d:SEAR:PEAK:POL NEG;", w727) -> (resulting string=w726:string)  [unwired: 2 in, 1 out]
            }
            frame "Both" {
              n232 = Format Into String(format string=":CALC:USER:TRAC7:MARK%d:SEAR:PEAK:POL BOTH;", w730) -> (resulting string=w729:string)  [unwired: 2 in, 1 out]
            }
          }
          n233 = Pick Line(multi-line string=":CALC:USER:TRAC7:ALLM:SEAR:DOM:Y BDM;\n:CALC:USER:TRAC7:ALLM:SEAR:DOM:Y FRAN;", line index=w699) -> (output string=w698:string)  [unwired: 1 in]
          n234 = Pick Line(multi-line string=":CALC:USER:TRAC7:ALLM:SEAR:DOM:X BDM;\n:CALC:USER:TRAC7:ALLM:SEAR:DOM:X FRAN;", line index=w702) -> (output string=w701:string)  [unwired: 1 in]
          n235 = Format Into String(format string="%.;:CALC:USER:TRAC7:MARK%d:SEAR:PEAK:EXC %g;\n%.;:CALC:USER:TRAC7:MARK%d:SEAR:TARG:Y %g;", w709, w708, w709, w707) -> (resulting string=w712:string)  [unwired: 2 in, 1 out]
          n236 = Concatenate Strings(w712, w711, w710, w701, w698) -> (w704:string)
        }
        frame 8 {
          # "Trace 8"
          n237 = case shown="\"Positive\", Default" w739 {
            tunnel: w743 -> [w750 w752 w755]
            tunnel: [w748 w751 w754] -> w744
            frame "Positive", Default {
              n238 = Format Into String(format string=":CALC:USER:TRAC8:MARK%d:SEAR:TARG:TRAN POS;", w750) -> (resulting string=w748:string)  [unwired: 2 in, 1 out]
            }
            frame "Negative" {
              n239 = Format Into String(format string=":CALC:USER:TRAC8:MARK%d:SEAR:TARG:TRAN NEG;", w752) -> (resulting string=w751:string)  [unwired: 2 in, 1 out]
            }
            frame "Both" {
              n240 = Format Into String(format string=":CALC:USER:TRAC8:MARK%d:SEAR:TARG:TRAN BOTH;", w755) -> (resulting string=w754:string)  [unwired: 2 in, 1 out]
            }
          }
          n241 = case shown="\"Positive\", Default" w740 {
            tunnel: w743 -> [w759 w761 w764]
            tunnel: [w757 w760 w763] -> w745
            frame "Positive", Default {
              n242 = Format Into String(format string=":CALC:USER:TRAC8:MARK%d:SEAR:PEAK:POL POS;", w759) -> (resulting string=w757:string)  [unwired: 2 in, 1 out]
            }
            frame "Negative" {
              n243 = Format Into String(format string=":CALC:USER:TRAC8:MARK%d:SEAR:PEAK:POL NEG;", w761) -> (resulting string=w760:string)  [unwired: 2 in, 1 out]
            }
            frame "Both" {
              n244 = Format Into String(format string=":CALC:USER:TRAC8:MARK%d:SEAR:PEAK:POL BOTH;", w764) -> (resulting string=w763:string)  [unwired: 2 in, 1 out]
            }
          }
          n245 = Pick Line(multi-line string=":CALC:USER:TRAC8:ALLM:SEAR:DOM:Y BDM;\n:CALC:USER:TRAC8:ALLM:SEAR:DOM:Y FRAN;", line index=w733) -> (output string=w732:string)  [unwired: 1 in]
          n246 = Pick Line(multi-line string=":CALC:USER:TRAC8:ALLM:SEAR:DOM:X BDM;\n:CALC:USER:TRAC8:ALLM:SEAR:DOM:X FRAN;", line index=w736) -> (output string=w735:string)  [unwired: 1 in]
          n247 = Format Into String(format string="%.;:CALC:USER:TRAC8:MARK%d:SEAR:PEAK:EXC %g;\n%.;:CALC:USER:TRAC8:MARK%d:SEAR:TARG:Y %g;", w743, w742, w743, w741) -> (resulting string=w746:string)  [unwired: 2 in, 1 out]
          n248 = Concatenate Strings(w746, w745, w744, w735, w732) -> (w738:string)
        }
      }
    }
  }
  n249 = VISA Write(VISA resource name="VISA resource name", write buffer=w8, error in (no error)="error in (no error)") -> (VISA resource name out=w7:refnum<visa-resource-name>, error out=w6:errorcluster)  [unwired: 1 out]
  n250 = call "Error Query.vi"("error in (no error)"=w6, "VISA resource name"=w7) -> ("error out"=→"error out":errorcluster, "VISA resource name out"=→"VISA resource name out":refnum<visa-resource-name>)  [unwired: 6 in, 2 out]
